vi "ws_users update current user header.vi"(8 "error in (no error)":errorcluster, 9 "Current User Changes? (f)":bool, 10 "new Current User":T1, 11 "httpRequestID":u32) -> (0 "error out":errorcluster)   [LabVIEW 2011]
uses:
  server/database/Users/User Record.ctl
  <vilib>/wsapi/subVIs/Write Single Session Variable.vi
  <vilib>/wsapi/NI_WebServices.lvlib
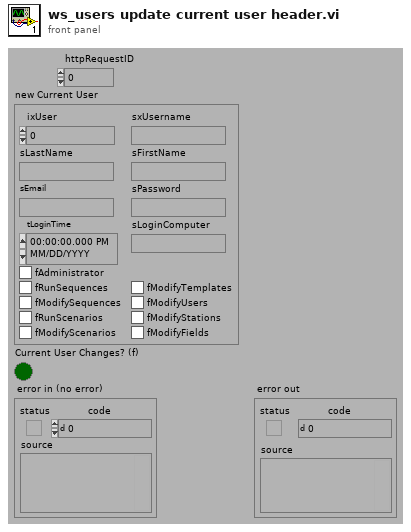
[diagram p1: front panel]
types:
  T1 = typedef "User Record.ctl" = cluster{"ixUser":i32, "sxUsername":string, "sLastName":string, "sFirstName":string, "sEmail":string, "sPassword":string, "tLoginTime":timestamp, "sLoginComputer":string, "fAdministrator":bool, "fRunSequences":bool, "fModifySequences":bool, "fRunScenarios":bool, "fModifyScenarios":bool, "fModifyTemplates":bool, "fModifyUsers":bool, "fModifyStations":bool, "fModifyFields":bool}
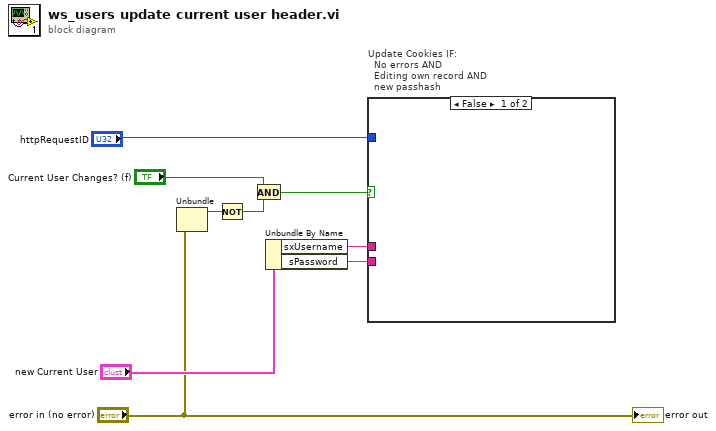
[diagram p0: block diagram]
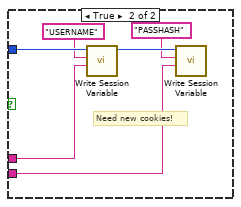
[diagram p2: hidden frame]
diagram:
  n1 = Unbundle("error in (no error)") -> ("status"=w5:bool)  [unwired: 2 out]
  n2 = Not(x=w5) -> (.not. x?=w4:bool)
  n3 = And(x="Current User Changes? (f)", y=w4) -> (x .and. y?=w6:bool)
  n4 = Unbundle By Name("new Current User") -> ("sxUsername"=w9:string, "sPassword"=w8:string)
  n5 = case "Update Cookies IF:\n  No errors AND\n  Editing own record AND\n  new passhash" shown="False" w6 {
    tunnel: "httpRequestID" -> [_ w15]
    tunnel: w9 -> [_ w13]
    tunnel: w8 -> [_ w10]
    frame False {
    }
    frame True {
      # "Need new cookies!"
      n6 = call-poly <vilib>:"Write Session Variable.vi"("value"=w13, "key"="USERNAME" ("cookie name"), "httpRequestID"=w15) -> ("httpRequestID out"=w12:u32)  [unwired: 5 in, 3 out]
      n7 = call-poly <vilib>:"Write Session Variable.vi"("value"=w10, "key"="PASSHASH" ("cookie name"), "httpRequestID"=w12) -> ()  [unwired: 5 in, 4 out]
    }
  }
  "error out" <- "error in (no error)"
